vi "ECG Data.vi"() -> (1 "Clean ECG":waveform(dbl), 3 "Noisy ECG":waveform(dbl))   [LabVIEW 2021]
doc: "Generate variable ECG Signal with Noise and return 1 second of data at 1 kHz, This VI will only return data once every second."
uses:
  <vilib>/ptbypt/NI_PtbyPt.lvlib
  <vilib>/Analysis/NI_AALBase.lvlib
panel:
  in  "Respiration (mV)":dbl=0.30000000000000004 step=0.01 format="%#_13g"
  in  "Power line noise (mV)":dbl=0.2 step=0.01 format="%#_13g"
  in  "Uniform noise (mV)":dbl=0.1 step=0.01 format="%#_13g"
  out "ECG Data":dbl[][](graph)
  in  "BPM":dbl=80.0
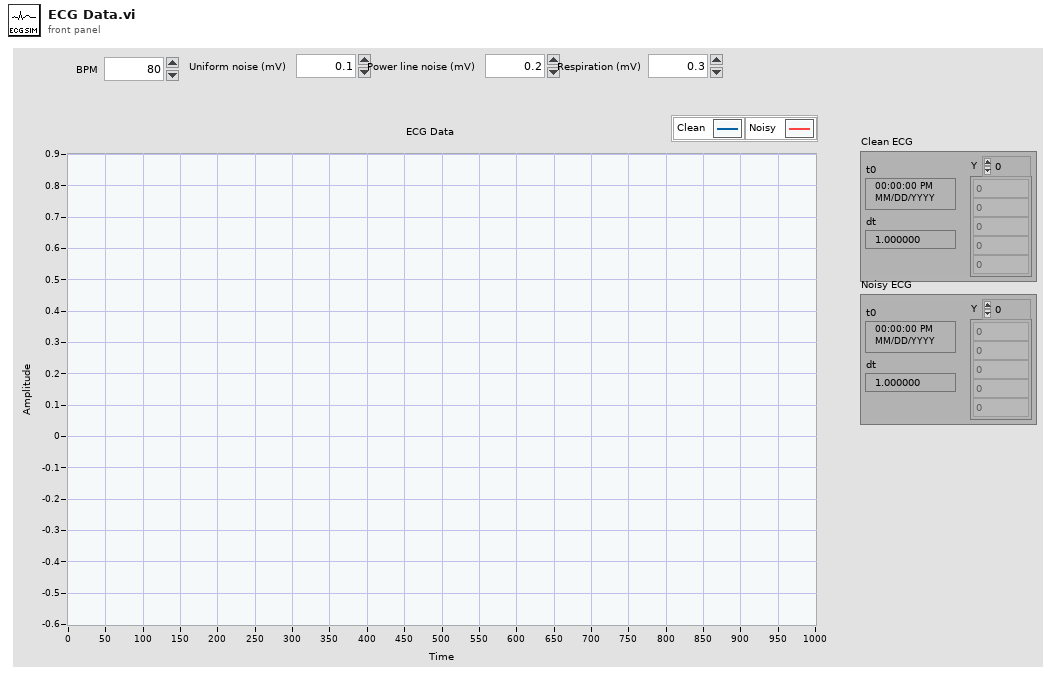
[diagram p1: front panel]
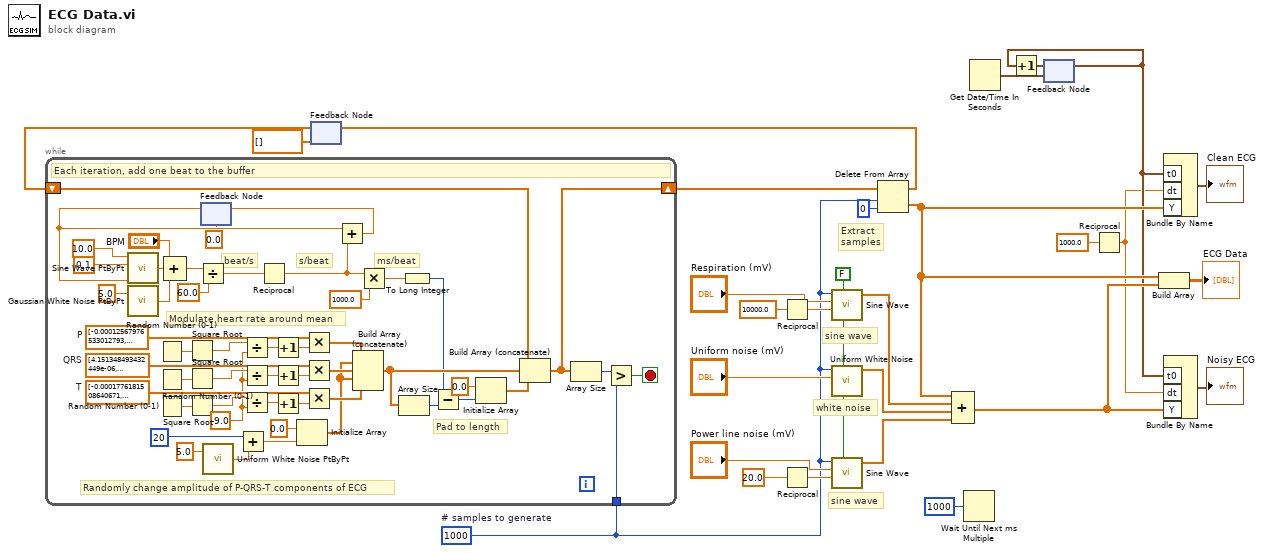
[diagram p0: block diagram]
diagram:
  w3 = 1000  # # samples to generate
  w19 = FALSE ("reset phase")
  # "white noise"
  # "sine wave"
  # "sine wave"
  # "Extract\nsamples"
  n1 = feedback #1(dbl[] [] ("result")) -> (w17:dbl[])
  n2 = while {
    shift-right: [w45] -> w16
    shift-left: w17 -> [w46]
    tunnel: w3 -> [w43]
    stop <- w42 stop-if-true
    w41 = dbl[] [-0.00012567976533012793, -0.0014694254768103366, -0.0017831669740602317, 0.0005521560370043469, 0.0056025916080220525, 0.012304630359609308, 0.019851099607961144, 0.02823674532089656, 0.03764100203655081, 0.04765888691840425, 0.05717782752542559, 0.06501117993393439, 0.07095750981965734, 0.0763752143854486, 0.08325643343279107, 0.0922470692091116, 0.10173304403381168, 0.10924086289853346, 0.11357356302731147, 0.11528582403391874, 0.11554144712995708, 0.11530946184902915, 0.11546176901781002, 0.11643903911022643, 0.11726047306235603, 0.11575502728253625, 0.11077228886216002, 0.1039101498477571, 0.09819113203508904, 0.09496148245546651, 0.09271835422032289, 0.0890935920541347, 0.08336372964787635, 0.07669420007325677, 0.07042320153125595, 0.06469751149548504, 0.05877602299559262, 0.052298089219977334, 0.046009457218010495, 0.041137769969732015, 0.03800344343862597, 0.03539191424774308, 0.031569751692377565, 0.02594964590617067, 0.01956024355950041, 0.013968045791526593, 0.010133975105964907, 0.008280344663257383, 0.008112958676124573, 0.00862879026533863, 0.008219096268210472, 0.005874584797364391, 0.0023887750964854734, -0.0002528841726185721, -0.0009039608099173942, -0.00026407387882808667, 0.00026671487534641583, 0.00018226194361497386, -5.286122401419127e-05, -4.6453219589199835e-05]  # P
    w65 = -9.0 ("y")
    w78 = dbl[] [-0.0001776181508640671, -0.0004630612116769867, 0.0003114215096199863, 0.0018439106337725553, 0.003120037302026467, 0.003963928118302236, 0.0051568072488554885, 0.006988112813270429, 0.008714712905824509, 0.009820698062247103, 0.010886921492989253, 0.012567761144433162, 0.01444305339714006, 0.015728430021992888, 0.016610617921724635, 0.017871888636150166, 0.019414045136419388, 0.020256357792424358, 0.02016441246822309, 0.020291211908610062, 0.021717971845624934, 0.024083102053686675, 0.026258404641084233, 0.02785551397634441, 0.029372582213258155, 0.0311788288826391, 0.033111761431868766, 0.035005260538266234, 0.03690357638481334, 0.03860424879022718, 0.03958031808455208, 0.03968762273020115, 0.03960013224328559, 0.04022165137397694, 0.04184716024960183, 0.044089813912890394, 0.04637036232480549, 0.04819619391656354, 0.04920526472076089, 0.049412330992148853, 0.049448701127021905, 0.05015897594734128, 0.05172813955031863, 0.05340152665089439, 0.054306928361134786, 0.05446901376405825, 0.05476271554066981, 0.0558433306536703, 0.05738018619420671, 0.058523840910811434, 0.058946238121618234, 0.05909425435607985, 0.05943148719975233, 0.059846702527595885, 0.06007894342399136, 0.06041703989444952, 0.06147876520694166, 0.06332259642208088, 0.06528866771414267, 0.06693657988198334, 0.06874055787449825, 0.07148498140905933, 0.0752116133097462, 0.07919629169887961, 0.08287185702895537, 0.08632542278288237, 0.08984730481420669, 0.09344285036623914, 0.09700010445739063, 0.10058194853001776, 0.10423112985866474, 0.10771822435549952, 0.11087148235043448, 0.11408445348727815, 0.1181077385635164, 0.12321835812241133, 0.12881433887025945, 0.1339433126242326, 0.13809489754288037, 0.14143146278350055, 0.14446545171906855, 0.14769784440922848, 0.15146379752991843, 0.15590507541996232, 0.161007546431198, 0.1666593442676438, 0.17259647822168875, 0.17827380773935556, 0.18302329353478672, 0.1866548426196393, 0.18990992887062752, 0.19398149030289766, 0.1993124149204629, 0.2049897757544247, 0.20964058339424926, 0.2129862508134024, 0.21623914679733627, 0.22075186810282146, 0.2264425407502295, 0.23188347575519053, 0.23596729172231004, 0.2391539396742993, 0.24286145595642084, 0.24785055579799467, 0.2535327929969536, 0.25877516700073344, 0.2629704865264248, 0.2661913560859642, 0.268680852950584, 0.27058947517381676, 0.272132660610728, 0.2736578409863852, 0.27542898157667806, 0.2774522278791817, 0.27951249778845316, 0.2812556797472632, 0.28230463370090464, 0.282574160764998, 0.2825647198097731, 0.28310543520218595, 0.284598116870691, 0.2865871391666439, 0.2881627629465082, 0.2886589740932761, 0.287909509707062, 0.28616122914371506, 0.28408792744693645, 0.2826647879231937, 0.2824380387874035, 0.2827729949851837, 0.2823047077415071, 0.2804823007901596, 0.2783660546118741, 0.27745631634350243, 0.27784920325770124, 0.2779955289836025, 0.27632996933377746, 0.27276025963457334, 0.2684303125811568, 0.2644089969379688, 0.26092894217694435, 0.25766726990093963, 0.25430247035827314, 0.25068215523613835, 0.24667309686579925, 0.24201492144836018, 0.23635646617451792, 0.2295590822526166, 0.2221073797531595, 0.21506670638887604, 0.20924633053544492, 0.20427477635896782, 0.1988144993116763, 0.1919850493603946, 0.18442712463672556, 0.17762884823482986, 0.17221252182406208, 0.16722431991755315, 0.16126230616887446, 0.1540486058585101, 0.14662909562352047, 0.1401540436815642, 0.13478785492642195, 0.12985587233133436, 0.1247371603195324, 0.11935227393413056, 0.11391338513512358, 0.10853929658325069, 0.1032274076818882, 0.09798615105000583, 0.0927840451646221, 0.08744898089959423, 0.08184519892089934, 0.07619039635683399, 0.07101809717272083, 0.06670820924471652, 0.06313601844896945, 0.05985486446142827, 0.05650706875054801, 0.05294757793826516, 0.049136202959804066, 0.045203073427345454, 0.041614287897776193, 0.038930427953916574, 0.0371727104234341, 0.03557874292645027, 0.0332130437752047, 0.029780769393755846, 0.025718042863403325, 0.0216342777703808, 0.01793900537013962, 0.014920560034791646, 0.01273561913239538, 0.011113590123419169, 0.00941124986320002, 0.007337248173744998, 0.005480380760557352, 0.0047015307636632244, 0.004956904273425134, 0.005102126257002021, 0.0040796190781224335, 0.0020741674517966227, 0.0002483963892362318, -0.0005222269721209833, -0.000376235243451864, -1.3213967704990478e-05, 0.00012229969433388073, 6.654899254664597e-05, 4.306958115056047e-06, -7.0556889872634645e-06]  # T
    w79 = dbl[] [4.151348493432449e-06, 5.151233507849264e-05, 0.00020774563593565094, 0.00038136512181582223, 0.0002167015988830232, -0.0007101282481652361, -0.002550268594680167, -0.005127672725239974, -0.00826859945821789, -0.012075932626889437, -0.016763023896099502, -0.022273803200951535, -0.028209812740556447, -0.034142649512473845, -0.03988453327002574, -0.04544584078753644, -0.05090987999880103, -0.056488682757594985, -0.0625804009816537, -0.06952245894662723, -0.07721788730959935, -0.08515719386964048, -0.09291112681050027, -0.10047834289678655, -0.10798299963456105, -0.1150870876036732, -0.12090576126040488, -0.12454898315652872, -0.12559873989029938, -0.12404394826899758, -0.12004691264253169, -0.11402394516557679, -0.10673095398925216, -0.09877469843053208, -0.08990978272069743, -0.07920637103887988, -0.06622946876564087, -0.05182078157745957, -0.03728233259628653, -0.02281692063855227, -0.007276487312661916, 0.010224859772952762, 0.028713705367761716, 0.04589992730094334, 0.06058210395491006, 0.07439157418809314, 0.09089512942351469, 0.11286873764953083, 0.14052886553725402, 0.17243593702518725, 0.207810179221354, 0.24754830909711803, 0.2930229848880155, 0.34446843252806325, 0.40088320893543083, 0.46100114309112816, 0.5235813312098516, 0.586785047961389, 0.6480507142721309, 0.7049624170898773, 0.7558373532371265, 0.799238907764192, 0.8334856593472695, 0.8571581219561719, 0.869725086456287, 0.8711101234613159, 0.8608772158949052, 0.8384040007914358, 0.8037276098838562, 0.7577987382529482, 0.702221776972642, 0.6392553786435752, 0.5714233169407696, 0.5000194537606367, 0.42455203924172724, 0.34546116753493944, 0.2672133483266096, 0.19580404604617505, 0.13160031252479876, 0.06750525050355274, -0.0017736081955658292, -0.06900891931355424, -0.11723655007286002, -0.13556263779812236, -0.130318688195673, -0.11866043553587563, -0.1127943885761295, -0.11270160909450093, -0.11248244651388464, -0.10935068025589967, -0.10496648965326359, -0.10103715994930484, -0.09675970301468258, -0.09031367444733192, -0.08102353281510948, -0.06977912618006636, -0.0583323236063952, -0.04836693651846715, -0.0405394587535137, -0.03420000578293978, -0.028386004176828503, -0.022984641331407693, -0.018514251966485536, -0.015039794622947193, -0.012014197225108913, -0.00914314724593922, -0.0066724039093382665, -0.004691476270506584, -0.0028551522384169256, -0.0010845350545890364, 7.95142286322358e-05, 0.00026259219759366124]  # QRS
    # "Modulate heart rate around mean"
    # "Pad to length"
    # "Randomly change amplitude of P-QRS-T components of ECG"
    # "ms/beat"
    # "s/beat"
    # "beat/s"
    # "Each iteration, add one beat to the buffer"
    n3 = call <vilib>:"Gaussian White Noise PtByPt.vi"("standard deviation"=5.0 ("amplitude")) -> ("Gaussian white noise"=w58:dbl)  [unwired: 2 in]
    n4 = Random Number (0-1)() -> (number: 0 to 1=w70:dbl)
    n5 = Random Number (0-1)() -> (number: 0 to 1=w72:dbl)
    n6 = Random Number (0-1)() -> (number: 0 to 1=w77:dbl)
    n7 = Square Root(x=w70) -> (sqrt(x)=w69:dbl)
    n8 = Square Root(x=w72) -> (sqrt(x)=w71:dbl)
    n9 = Square Root(x=w77) -> (sqrt(x)=w66:dbl)
    n10 = feedback #2(0.0) -> (w33:dbl)
    n11 = call <vilib>:"Sine Wave PtByPt.vi"("time"=w33, "frequency"=0.1, "amplitude"=10.0) -> ("sine wave"=w35:dbl)  [unwired: 1 in]
    n12 = Compound Arithmetic op=ADD("BPM", w35, w58) -> (w56:dbl)
    n13 = Divide(x=w56, y=60.0) -> (x/y=w57:dbl)
    n14 = call <vilib>:"Uniform White Noise PtByPt.vi"("amplitude"=5.0) -> ("uniform white noise"=w40:dbl)  [unwired: 2 in]
    n15 = Add(x=20 ("dimension size"), y=w40) -> (x+y=w37:dbl)
    n16 = Divide(x=w69, y=w65) -> (x/y=w68:dbl)
    n17 = Divide(x=w71, y=w65) -> (x/y=w74:dbl)
    n18 = Divide(x=w66, y=w65) -> (x/y=w76:dbl)
    n19 = Reciprocal(x=w57) -> (1/x=w31:dbl)
    n20 = Increment(x=w68) -> (x+1=w67:dbl)
    n21 = Increment(x=w74) -> (x+1=w73:dbl)
    n22 = Increment(x=w76) -> (x+1=w75:dbl)
    n23 = Initialize Array(0.0 ("element"), w37) -> (w60:dbl[])
    n24 = Multiply(x=w41, y=w67) -> (x*y=w64:dbl[])
    n25 = Multiply(x=w79, y=w73) -> (x*y=w63:dbl[])
    n26 = Multiply(x=w78, y=w75) -> (x*y=w62:dbl[])
    n27 = Add(x=w33, y=w31) -> (x+y=w32:dbl)
    n28 = feedback-in #2(w32) -> ()
    n29 = Build Array (concatenate)(w64, w60, w63, w60, w62) -> (w50:dbl[])
    n30 = Multiply(x=w31, y=1000.0) -> (x*y=w48:dbl)
    n31 = Array Size(array=w50) -> (size(s)=w53:i32)
    n32 = To Long Integer(number=w48) -> (32bit integer=w49:i32)
    n33 = Subtract(x=w49, y=w53) -> (x-y=w54:i32)
    n34 = Initialize Array(0.0 ("element"), w54) -> (w52:dbl[])
    n35 = Build Array (concatenate)(w46, w50, w52) -> (w45:dbl[])
    n36 = Array Size(array=w45) -> (size(s)=w44:i32)
    n37 = Greater?(x=w44, y=w43) -> (0:w42:bool)
  }
  n38 = Reciprocal(x=10000.0 ("frequency")) -> (1/x=w21:dbl)
  n39 = Reciprocal(x=20.0 ("frequency")) -> (1/x=w26:dbl)
  n40 = call <vilib>:"Sine Wave.vi"("samples"=w3, "amplitude"="Respiration (mV)", "frequency"=w21, "reset phase"=w19) -> ("sine wave"=w22:dbl[])  [unwired: 1 in, 2 out]
  n41 = call <vilib>:"Uniform White Noise.vi"("initialize?"=w19, "amplitude"="Uniform noise (mV)", "samples"=w3) -> ("uniform white noise"=w1:dbl[])  [unwired: 7 in, 1 out]
  n42 = call <vilib>:"Sine Wave.vi"("samples"=w3, "amplitude"="Power line noise (mV)", "frequency"=w26, "reset phase"=w19) -> ("sine wave"=w20:dbl[])  [unwired: 1 in, 2 out]
  n43 = Delete From Array(array=w16, length=w3, index=0) -> (deleted portion=w12:dbl[], array with subset deleted=w14:dbl[])
  n44 = feedback-in #1(w14) -> ()
  n45 = Compound Arithmetic op=ADD(w12, w22, w1, w20) -> (w11:dbl[])
  n46 = Wait Until Next ms Multiple(millisecond multiple=u32 1000) -> ()  [unwired: 1 out]
  n47 = Get Date/Time In Seconds() -> (seconds since 1Jan1904=w10:timestamp)
  n48 = feedback #3(w10) -> (w7:timestamp)
  n49 = Increment(x=w7) -> (x+1=w9:timestamp)
  n50 = feedback-in #3(w9) -> ()
  n51 = Reciprocal(x=1000.0 ("frequency")) -> (1/x=w6:dbl)
  n52 = Build Array(w12, w11) -> (→"ECG Data":dbl[][])
  n53 = Bundle By Name("t0"=w7, "dt"=w6, "Y"=w12) -> (→"Clean ECG":waveform(dbl))  [unwired: 1 in]
  n54 = Bundle By Name("t0"=w7, "dt"=w6, "Y"=w11) -> (→"Noisy ECG":waveform(dbl))  [unwired: 1 in]
